vi "wait_with_status.vi"(4 "stat ref":refnum<vi>, 6 "stop ref":refnum<vi>, 8 "error in":errorcluster, 9 "comment":string, 10 "ignore error (False)":bool, 11 "ms to wait":i32) -> (0 "error out":errorcluster)   [LabVIEW 2013, in "varilib.lvlib"]
doc: "Interruptable delay timer. It waits for given amount of milliseconds. When 'stop ref' is assigned with reference to boolean button it will terminate the delay when logical state of the boolean is True. If 'stat ref' is assigned with reference to string indicator and delay is over 1 second it will periodically write status string in following format:'Waiting 3 of 10 seconds%s' where %s is content of 'comment' input. When the wait loop is done the original content of 'stat ref' will be restored."
uses:
  varilib.lvlib
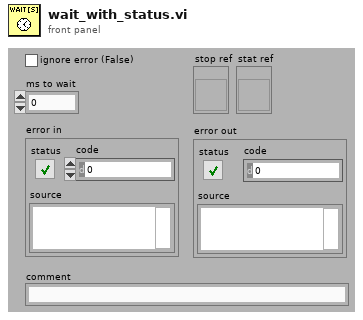
[diagram p1: front panel]
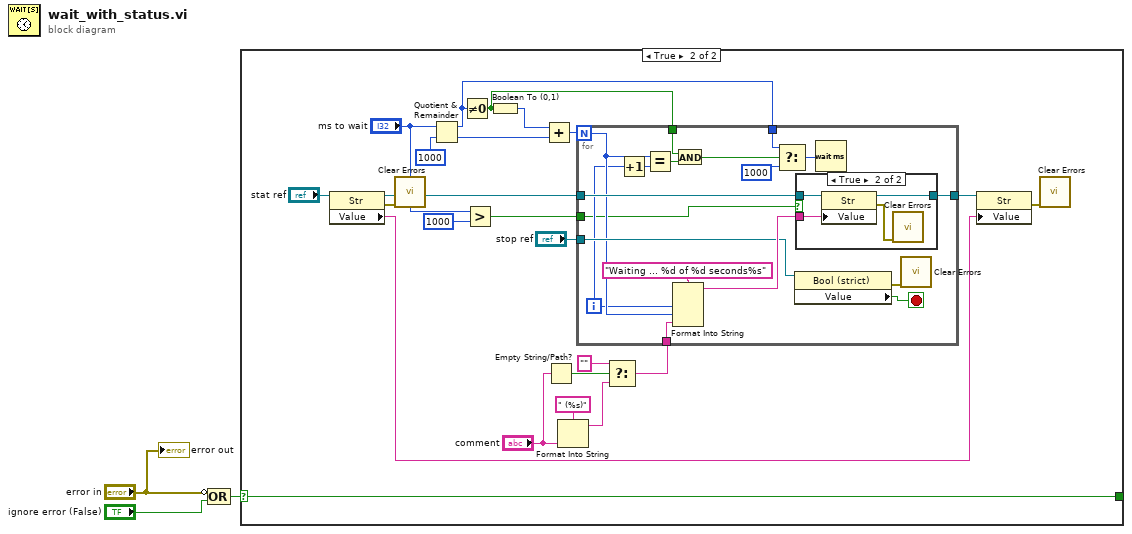
[diagram p0: block diagram]
diagram:
  n1 = Compound Arithmetic op=OR(invert "error in", "ignore error (False)") -> (w1:bool)
  n2 = case shown="True" w1 {
    selector: w1 -> [w4 w11]
    tunnel: [w4 w11] -> _
    frame False {
    }
    frame True {
      n3 = property class="Str"(reference="stat ref") -> (reference out=w9:refnum<vi>, error out=w8:errorcluster, "Value"=w5:string)  [unwired: 1 in]
      n4 = call <vilib>:"Clear Errors.vi"("error in (no error)"=w8) -> ()  [unwired: 6 in, 1 out]
      n5 = Quotient & Remainder(x="ms to wait", y=1000) -> (x-y*floor(x/y)=w17:i32, floor(x/y)=w18:i32)
      n6 = Not Equal To 0?(x=w17) -> (x != 0?=w16:bool)
      n7 = Greater?(x="ms to wait", y=1000) -> (0:w12:bool)
      n8 = Boolean To (0,1)(Boolean=w16) -> (0, 1=w15:i16)
      n9 = Add(x=w15, y=w18) -> (x+y=w19:i32)
      n10 = Empty String/Path?(string/path="comment") -> (empty?=w25:bool)
      n11 = Format Into String(format string=" (%s)", "comment") -> (resulting string=w22:string)  [unwired: 2 in, 1 out]
      n12 = Select(t="", s=w25, f=w22) -> (s? t:f=w24:string)
      n13 = for {
        N: w19 -> [w36]
        tunnel: w9 -> [w45]
        tunnel: "stop ref" -> [w42]
        tunnel: w24 -> [w40]
        tunnel: w17 -> [w37]
        tunnel: w16 -> [w32]
        tunnel: w12 -> [w30]
        tunnel: [w28] -> w7
        i -> [w34]
        stop <- w41 stop-if-true
        n14 = Increment(x=w34) -> (x+1=w35:i32)
        n15 = Equal?(x=w36, y=w35) -> (x = y?=w33:bool)
        n16 = Format Into String(format string="Waiting ... %d of %d seconds%s", w34, w36, w40) -> (resulting string=w44:string)  [unwired: 2 in, 1 out]
        n17 = And(x=w32, y=w33) -> (x .and. y?=w31:bool)
        n18 = Select(t=w37, s=w31, f=u32 1000 ("milliseconds to wait")) -> (s? t:f=w39:u32)
        n19 = property class="Bool (strict)"(reference=w42) -> (error out=w29:errorcluster, "Value"=w41:bool)  [unwired: 1 in, 1 out]
        n20 = case shown="True" w30 {
          tunnel: w45 -> [w46 w50]
          tunnel: w44 -> [_ w49]
          tunnel: [w46 w47] -> w28
          frame False {
          }
          frame True {
            n21 = property class="Str"(reference=w50, "Value"=w49) -> (reference out=w47:refnum<vi>, error out=w48:errorcluster)  [unwired: 1 in]
            n22 = call <vilib>:"Clear Errors.vi"("error in (no error)"=w48) -> ()  [unwired: 6 in, 1 out]
          }
        }
        n23 = Wait (ms)(milliseconds to wait=w39) -> ()  [unwired: 1 out]
        n24 = call <vilib>:"Clear Errors.vi"("error in (no error)"=w29) -> ()  [unwired: 6 in, 1 out]
      }
      n25 = property class="Str"(reference=w7, "Value"=w5) -> (error out=w6:errorcluster)  [unwired: 1 in, 1 out]
      n26 = call <vilib>:"Clear Errors.vi"("error in (no error)"=w6) -> ()  [unwired: 6 in, 1 out]
    }
  }
  "error out" <- "error in"
